vi "EQC mergeEQs.vi"() -> (0 "Error tick":bool)   [LabVIEW 2015, in "VIPM2.lvlib"]
doc: "Open a new window to run the EQs merging."
uses:
  VIPM2.lvlib
panel:
  in  "Cancel Button":bool
  in  "MERGE Button":bool
  in  "EQ Leak3 folder path":path caption="Leakage 3 EQ"
  in  "EQ Leak2 folder path":path caption="Leakage 2 EQ"
  in  "EQ Leak1 folder path":path caption="Leakage 1 EQ"
  in  "EQ Leak0 folder path":path caption="Leakage 0 EQ"
  # "Load Equalizations to merge"
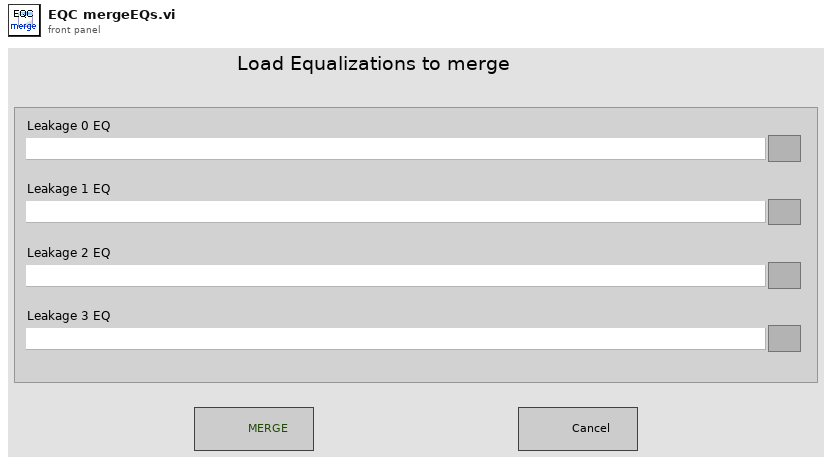
[diagram p1: front panel]
types:
  T1 = enum16{"open", "replace", "create", "open or create", "replace or create", "replace or create with confirmation"}
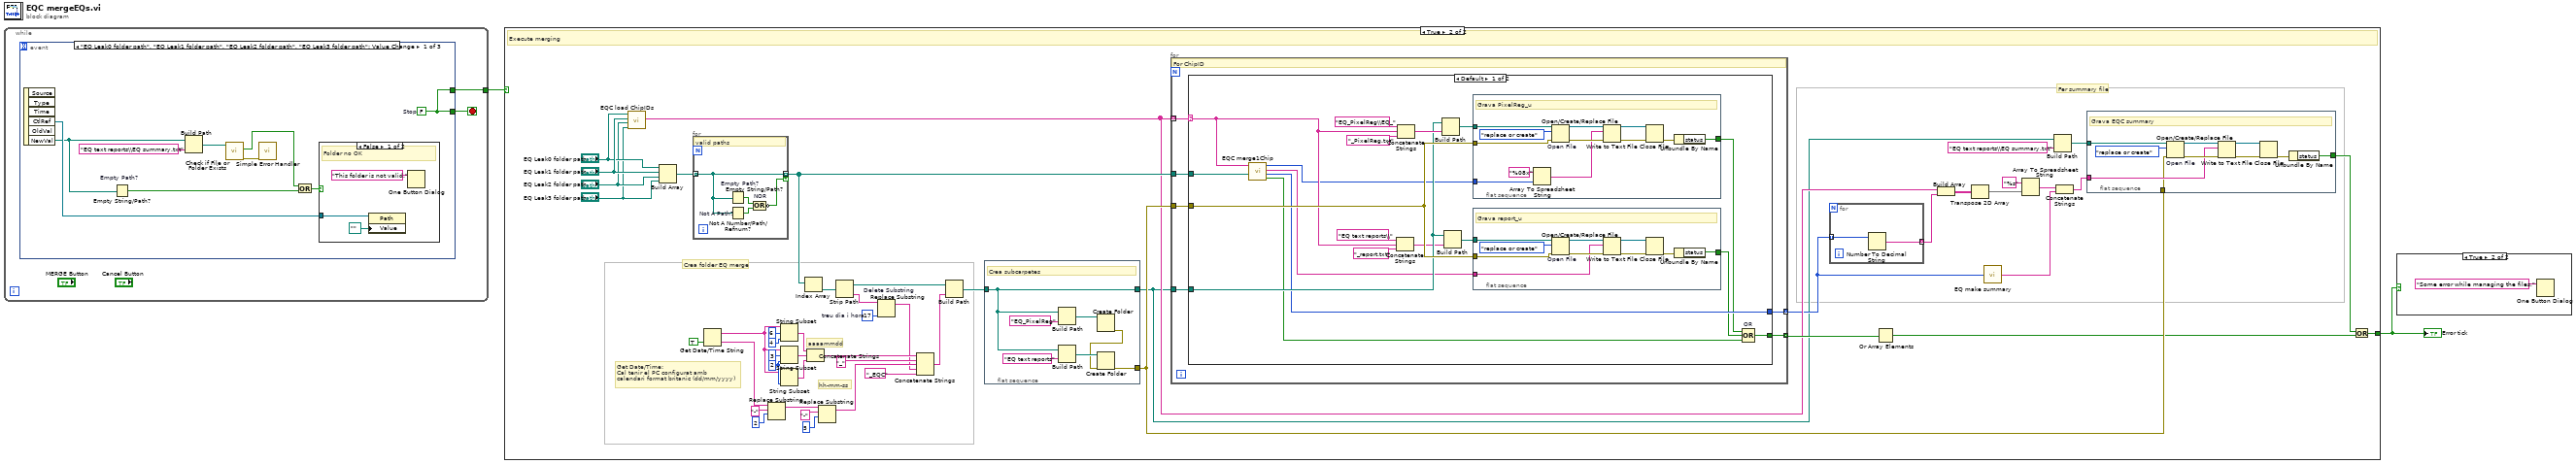
[diagram p0: block diagram]
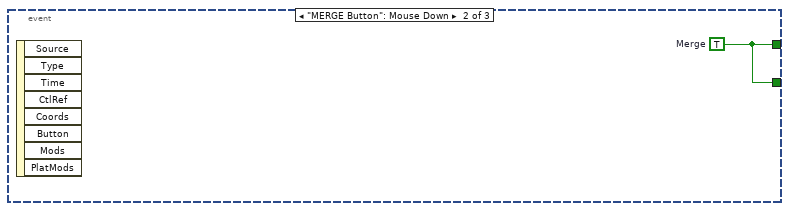
[diagram p4: hidden frame]
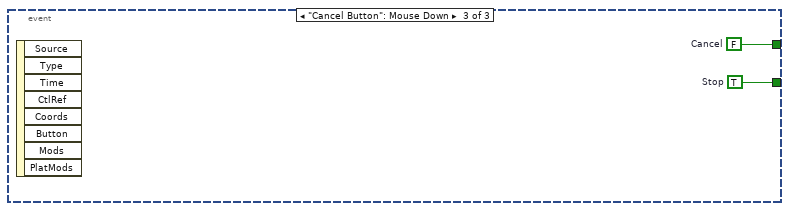
[diagram p5: hidden frame]
diagram:
  n1 = while {
    tunnel: [w3] -> w2
    stop <- w4 stop-if-true
    n2 = event shown="[0] \"EQ Leak0 folder path\", \"EQ Leak1 folder path\", \"EQ Leak2 folder path\", \"EQ Leak3 folder path\": Value Change" {
      selector: _ -> [_ _ _]
      dyn-events: _ -> [_ _ _]
      timeout: _ -> [_ _ _]
      tunnel: [w12 w17 w18] -> w4
      tunnel: [w12 w17 w19] -> w3
      event "EQ Leak0 folder path", "EQ Leak1 folder path", "EQ Leak2 folder path", "EQ Leak3 folder path": Value Change {
        w12 = FALSE  # Stop
        n3 = event-data() -> ("CtlRef"=w13:refnum<vi>, "NewVal"=w9:path)  [unwired: 1 in, 4 out]
        n4 = Empty String/Path? "Empty Path?"(string/path=w9) -> (empty?=w11:bool)
        n5 = Build Path(base path=w9, name or relative path="EQ text reports\\EQ summary.txt") -> (appended path=w7:path)
        n6 = call <vilib>:"Check if File or Folder Exists.vi"("path"=w7) -> ("error out"=w6:errorcluster, "file or folder exists?"=w5:bool)  [unwired: 8 in, 1 out]
        n7 = call <vilib>:"Simple Error Handler.vi"("error in (no error)"=w6) -> ()  [unwired: 4 in, 5 out]
        n8 = Or(x=w5, y=w11) -> (x .or. y?=w10:bool)
        n9 = case shown="False" w10 {
          tunnel: w13 -> [w15 _]
          frame False {
            # "Folder no OK"
            n10 = property class="Path"(reference=w15, "Value"=path "") -> ()  [unwired: 1 in, 2 out]
            n11 = One Button Dialog(message="This folder is not valid.") -> ()  [unwired: 1 in, 1 out]
          }
          frame True {
            # "Folder OK"
          }
        }
      }
      event "MERGE Button": Mouse Down {
        w17 = TRUE  # Merge
        n12 = event-data() -> ()  [unwired: 1 in, 8 out]
      }
      event "Cancel Button": Mouse Down {
        w18 = TRUE  # Stop
        w19 = FALSE  # Cancel
        n13 = event-data() -> ()  [unwired: 1 in, 8 out]
      }
    }
  }
  n14 = case shown="True" w2 {
    tunnel: [_ w22] -> w1
    frame False {
      # "Cancel"
    }
    frame True {
      w51 = 2 ("length (rest)")
      w58 = 17  # treu dia i hora
      # "Fer summary file"
      # "Crea folder EQ merge"
      # "Get Date/Time:\nCal tenir el PC configurat amb\ncalendari format britanic (dd/mm/yyyy)"
      # "hh-mm-ss"
      # "aaaammdd"
      # "Execute merging"
      n15 = call "EQC load ChipIDs.vi"("EQ Leak3 folder path"="EQ Leak3 folder path", "EQ Leak2 folder path"="EQ Leak2 folder path", "EQ Leak1 folder path"="EQ Leak1 folder path", "EQ Leak0 folder path"="EQ Leak0 folder path") -> ("ChipID list 1i2"=w35:string[])  [unwired: 7 in]
      n16 = Build Array "Build Array"("EQ Leak0 folder path", "EQ Leak1 folder path", "EQ Leak2 folder path", "EQ Leak3 folder path") -> (w62:path[])
      n17 = for {
        tunnel: w62 -> [w89] mode=indexing
        tunnel: [w89] -> w61 mode=indexing if=w88
        # "valid paths"
        n18 = Empty String/Path? "Empty Path?"(string/path=w89) -> (empty?=w91:bool)
        n19 = Not A Number/Path/Refnum? "Not A Path?"(number/path/refnum=w89) -> (NaN/Path/Refnum?=w90:bool)
        n20 = Compound Arithmetic op=OR "NOR"(w91, w90) -> (invert w88:bool)
      }
      n21 = Get Date/Time String(want seconds? (F)=TRUE) -> (date string=w50:string, time string=w55:string)  [unwired: 2 in]
      n22 = Replace Substring(3:2 ("offset (0)"), 4:"-" ("substring (\"\")"), 5:w55) -> (1:w45:string)  [unwired: 1 in, 1 out]
      n23 = String Subset(string=w50, offset (0)=6, length (rest)=4 ("length (rest)")) -> (substring=w52:string)
      n24 = String Subset(string=w50, offset (0)=3, length (rest)=w51) -> (substring=w53:string)
      n25 = String Subset(string=w50, length (rest)=w51) -> (substring=w54:string)  [unwired: 1 in]
      n26 = Index Array "Index Array"(array=w61) -> (element=w60:path)  [unwired: 1 in]
      n27 = Concatenate Strings(w52, w53, w54) -> (w42:string)
      n28 = Replace Substring(3:5 ("offset (0)"), 4:"-" ("substring (\"\")"), 5:w45) -> (1:w40:string)  [unwired: 1 in, 1 out]
      n29 = Strip Path(path=w60) -> (stripped path=w38:path, name=w59:string)
      n30 = Replace Substring "Delete Substring"(2:w58, 5:w59) -> (1:w39:string)  [unwired: 2 in, 1 out]
      n31 = Concatenate Strings "Concatenate Strings"(w42, "_" ("string"), w40, w39, "_EQC" ("string")) -> (w37:string)
      n32 = Build Path(base path=w38, name or relative path=w37) -> (appended path=w21:path)
      n33 = flat-sequence {
        tunnel: w21 -> [w71]
        tunnel: [w71] -> w20
        tunnel: [w69] -> w68
        frame #0 {
          # "Crea subcarpetes"
          n34 = Build Path(base path=w71, name or relative path="EQ_PixelReg") -> (appended path=w74:path)
          n35 = Build Path(base path=w71, name or relative path="EQ text reports") -> (appended path=w73:path)
          n36 = Create Folder(path (use dialog)=w74) -> (error out=w70:errorcluster)  [unwired: 2 in, 2 out]
          n37 = Create Folder(path (use dialog)=w73, error in=w70) -> (error out=w69:errorcluster)  [unwired: 1 in, 2 out]
        }
      }
      n38 = for {
        tunnel: w35 -> [w97] mode=indexing
        tunnel: w61 -> [w96]
        tunnel: w20 -> [w95]
        tunnel: [w94] -> w30 mode=indexing
        tunnel: [w93] -> w67 mode=indexing
        tunnel: w68 -> [w92]
        # "For ChipID"
        n39 = case shown="Default" w97 {
          selector: w97 -> [w106 _]
          tunnel: w96 -> [w115 _]
          tunnel: w95 -> [w109 _]
          tunnel: [w102 _] -> w94
          tunnel: [w98 _] -> w93
          tunnel: w92 -> [w116 _]
          frame Default {
            n40 = call "EQC merge1Chip.vi"("EQ Leak# folder paths"=w115, "ChipID"=w106) -> ("Error tick"=w99:bool, "quants GOOD"=w102:u8, "Merged report"=w103:string, "Merged PixelReg"=w104:u32[])  [unwired: 6 in]
            n41 = Concatenate Strings("EQ text reports\\" ("string"), w106, "_report.txt" ("string")) -> (w105:string)
            n42 = Concatenate Strings("EQ_PixelReg\\EQ_" ("string"), w106, "_PixelReg.txt" ("string")) -> (w111:string)
            n43 = Build Path(base path=w109, name or relative path=w111) -> (appended path=w112:path)
            n44 = Build Path(base path=w109, name or relative path=w105) -> (appended path=w110:path)
            n45 = flat-sequence {
              tunnel: w112 -> [w134]
              tunnel: [w131] -> w101
              tunnel: w104 -> [w129]
              tunnel: w116 -> [w127]
              frame #0 {
                # "Grava PixelReg_u"
                n46 = Array To Spreadsheet String(array=w129, 3:"%08x" ("format string")) -> (spreadsheet string=w128:string)  [unwired: 1 in]
                n47 = Open/Create/Replace File "Open File"(file path (use dialog)=w134, error in=w127, operation (0:open)=T1."replace or create") -> (refnum out=w138:refnum<file>, error out=w137:errorcluster)  [unwired: 3 in, 1 out]
                n48 = Write to Text File(file (use dialog)=w138, text=w128, error in=w137) -> (refnum out=w136:refnum<file>, error out=w135:errorcluster)  [unwired: 1 in, 1 out]
                n49 = Close File(refnum=w136, error in=w135) -> (error out=w132:errorcluster)  [unwired: 1 out]
                n50 = Unbundle By Name(w132) -> ("status"=w131:bool)
              }
            }
            n51 = flat-sequence {
              tunnel: w110 -> [w122]
              tunnel: [w119] -> w100
              tunnel: w103 -> [w118]
              tunnel: w116 -> [w117]
              frame #0 {
                # "Grava report_u"
                n52 = Open/Create/Replace File "Open File"(file path (use dialog)=w122, error in=w117, operation (0:open)=T1."replace or create") -> (refnum out=w126:refnum<file>, error out=w125:errorcluster)  [unwired: 3 in, 1 out]
                n53 = Write to Text File(file (use dialog)=w126, text=w118, error in=w125) -> (refnum out=w124:refnum<file>, error out=w123:errorcluster)  [unwired: 1 in, 1 out]
                n54 = Close File(refnum=w124, error in=w123) -> (error out=w120:errorcluster)  [unwired: 1 out]
                n55 = Unbundle By Name(w120) -> ("status"=w119:bool)
              }
            }
            n56 = Compound Arithmetic op=OR "OR"(w101, w100, w99) -> (w98:bool)
          }
          frame "0000" {
          }
        }
      }
      n57 = for {
        tunnel: w30 -> [w87] mode=indexing
        tunnel: [w86] -> w34 mode=indexing
        n58 = Number To Decimal String(number=w87) -> (decimal integer string=w86:string)  [unwired: 1 in]
      }
      n59 = Or Array Elements(Boolean array=w67) -> (logical OR=w24:bool)
      n60 = Build Array "Build Array"(w35, w34) -> (w33:string[][])
      n61 = Transpose 2D Array(2D array=w33) -> (transposed array=w32:string[][])
      n62 = call "EQ make summary.vi"("quants pixels bons per Chip"=w30) -> ("summary EQ"=w28:string)  [unwired: 4 in]
      n63 = Array To Spreadsheet String(array=w32, 3:"%s" ("format string")) -> (spreadsheet string=w29:string)  [unwired: 1 in]
      n64 = Build Path(base path=w20, name or relative path="EQ text reports\\EQ summary.txt") -> (appended path=w27:path)
      n65 = Concatenate Strings(w29, w28) -> (w25:string)
      n66 = flat-sequence {
        tunnel: w27 -> [w81]
        tunnel: [w78] -> w23
        tunnel: w25 -> [w77]
        tunnel: w68 -> [w76]
        frame #0 {
          # "Grava EQC summary"
          n67 = Open/Create/Replace File "Open File"(file path (use dialog)=w81, error in=w76, operation (0:open)=T1."replace or create") -> (refnum out=w85:refnum<file>, error out=w84:errorcluster)  [unwired: 3 in, 1 out]
          n68 = Write to Text File(file (use dialog)=w85, text=w77, error in=w84) -> (refnum out=w83:refnum<file>, error out=w82:errorcluster)  [unwired: 1 in, 1 out]
          n69 = Close File(refnum=w83, error in=w82) -> (error out=w79:errorcluster)  [unwired: 1 out]
          n70 = Unbundle By Name(w79) -> ("status"=w78:bool)
        }
      }
      n71 = Or(x=w23, y=w24) -> (x .or. y?=w22:bool)
    }
  }
  "Error tick" <- w1
  n72 = case shown="True" w1 {
    frame False {
    }
    frame True {
      n73 = One Button Dialog(message="Some error while managing the files.") -> ()  [unwired: 1 in, 1 out]
    }
  }
